vi "Climb Execute.vi"   [LabVIEW 2016]
uses:
  Climb Globals.vi
types:
  T1 = typedef "WPI_MotorControlDeviceRef.ctl" = cluster{"DeviceStatus":errorcluster, "Type":T2, "PWM":cluster{"PWM Channel":T3, "DeadBand":T4}, "CAN":cluster{"Device Number":u8, "SetOutput VI Ref":variant, "GetOutput VI Ref":variant, "Enable VI Ref":variant, "Disable VI Ref":variant, "Data":variant}, "Invert":bool}
  T2 = typedef "WPI_MotorControlType.ctl" = enum16{"PWM", "CAN"}
  T3 = typedef "FPGA_DIOPWMChannel.ctl" = enum8{"PWM 0", "PWM 1", "PWM 2", "PWM 3", "PWM 4", "PWM 5", "PWM 6", "PWM 7", "PWM 8", "PWM 9", "PWM MXP 0", "PWM MXP 1", "PWM MXP 2", "PWM MXP 3", "PWM MXP 4", "PWM MXP 5", "PWM MXP 6", "PWM MXP 7", "PWM MXP 8", "PWM MXP 9", "Invalid"}
  T4 = typedef "WPI_PWMDeadband.ctl" = cluster{"Name":string, "maxPositivePwm":i32, "minPositivePwm":i32, "centerPwm":i32, "maxNegativePwm":i32, "minNegativePwm":i32, "angularRange":u16}
  T5 = typedef "Climb Notifier.ctl" = cluster{"Up":bool, "Down":bool, "Climb Control List":T6}
  T6 = typedef "Climb Control Type.ctl" = enum16{"No Op", "Up", "Down"}
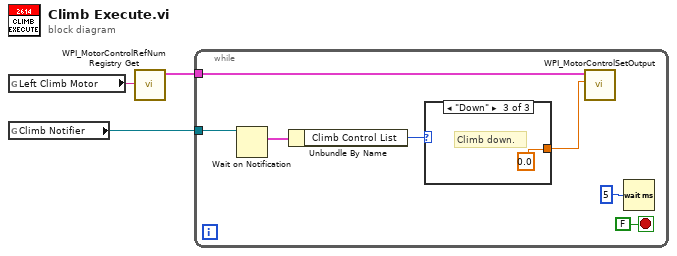
[diagram p0: block diagram]
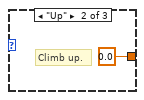
[diagram p3: hidden frame]
diagram:
  n1 = global read "Climb Globals.vi" "Left Climb Motor"() -> (w2:string)
  n2 = global read "Climb Globals.vi" "Climb Notifier"() -> (w1:refnum<notifier>)
  n3 = call <vilib>:"WPI_MotorControlRefNum Registry Get.vi"("refnum name"=w2) -> ("MotorControlDevRef"=w3:T1)  [unwired: 9 in, 1 out]
  n4 = while {
    tunnel: w1 -> [w7]
    tunnel: w3 -> [w6]
    stop <- FALSE stop-if-true
    n5 = Wait on Notification(notifier=w7) -> (notification=w8:T5)  [unwired: 3 in, 3 out]
    n6 = Unbundle By Name(w8) -> ("Climb Control List"=w5:T6)
    n7 = case shown="\"Down\"" w5 {
      tunnel: [_ 0.0 0.0] -> w4
      frame "No Op", Default {
      }
      frame "Up" {
        # "Climb up."
      }
      frame "Down" {
        # "Climb down."
      }
    }
    n8 = call <vilib>:"WPI_MotorControlSetOutput.vi"("Output"=w4, "MotorControlDevRef"=w6) -> ()  [unwired: 7 in, 3 out]
    n9 = Wait (ms)(milliseconds to wait=u32 5) -> ()  [unwired: 1 out]
  }
